vi "HatchManipulatorStateMachine.vi"(5 "Reset":bool, 6 "Place Release":bool, 7 "Floor Intake":bool, 8 "Place":bool, 9 "Slide/ No slide":bool, 10 "Feeder Station Intake":bool) -> (0 "Grip":bool, 1 "Hatch Manipulator State":T1, 2 "Extend":bool, 3 "Slide":bool)   [LabVIEW 2018]
uses:
  TypeDefs/HatchManipulatorState.ctl
  ArgosLib/Signal Processing/TypeDefs/EdgeDetector_Type.ctl
  ArgosLib/ArgosLib.lvlib
panel:
  in  "Grip Time (ms)":u32=500
  in  "Extend Time (ms)":u32=500
  in  "Slide Time (ms)":u32=500
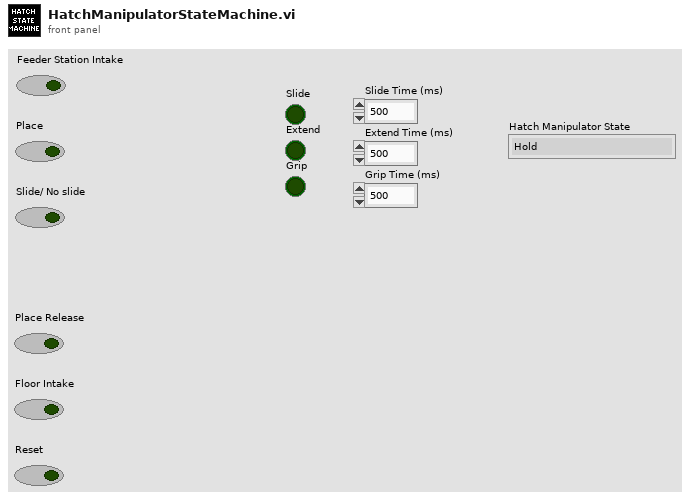
[diagram p1: front panel]
types:
  T1 = typedef "HatchManipulatorState.ctl" = enum16{"Hold", "Feeder Station Slide Out", "Feeder Station Slide Extend", "Feeder Station Slide Fully Extend", "Feeder Station Slide Grip", "Feeder Station Slide Retract", "Feeder Station Extend", "Feeder Station Fully Extended", "Feeder Station Grip", "Place Slide Out", "Place Slide Extend", "Place Slide Release", "Place Slide Retract", "Place Extend", "Place Release", "Place Retract", "Floor Intake Extend", "Floor Intake Grip"}
  T2 = typedef "ArgosLib.lvlib/EdgeDetector_Type.ctl" = enum16{"RisingEdge", "FallingEdge", "Both"}
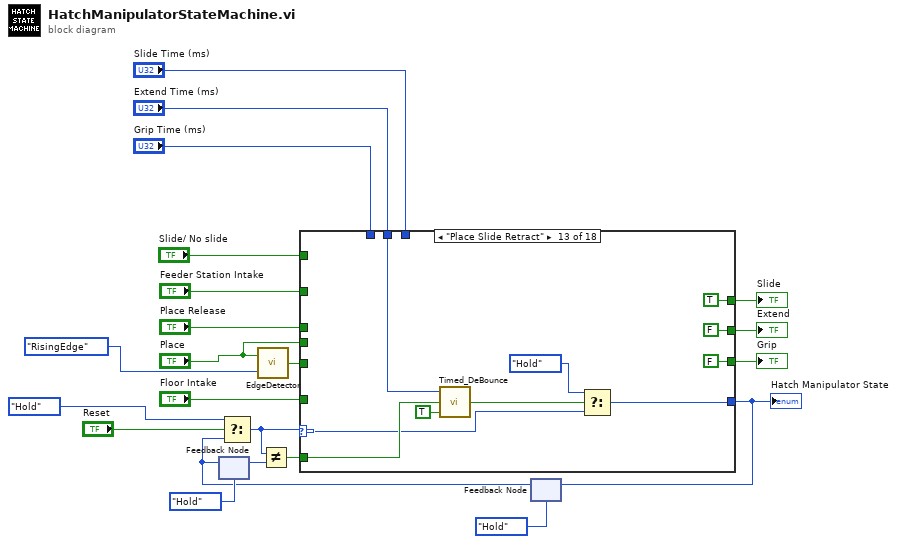
[diagram p0: block diagram]
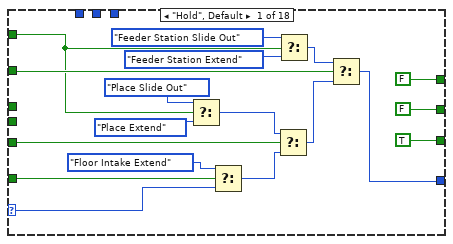
[diagram p2: hidden frame]
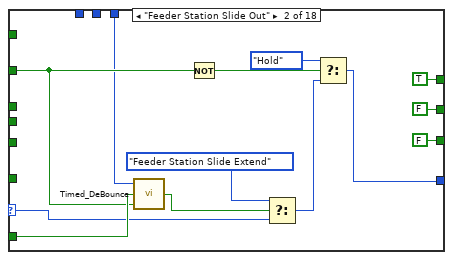
[diagram p3: hidden frame]
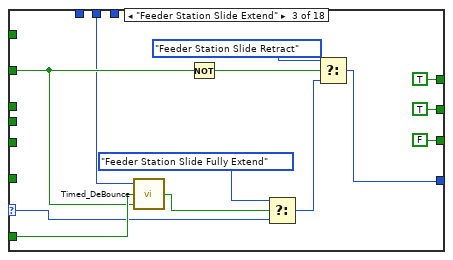
[diagram p4: hidden frame]
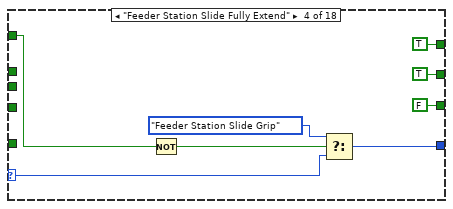
[diagram p5: hidden frame]
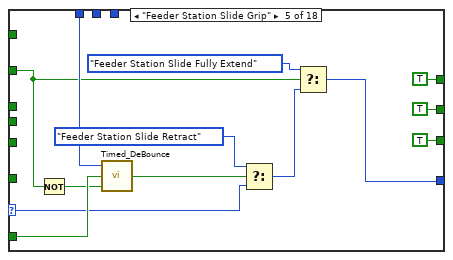
[diagram p6: hidden frame]
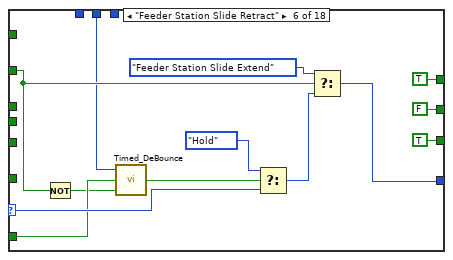
[diagram p7: hidden frame]
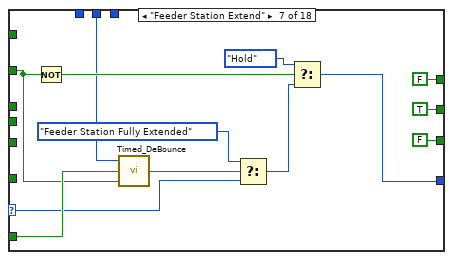
[diagram p8: hidden frame]
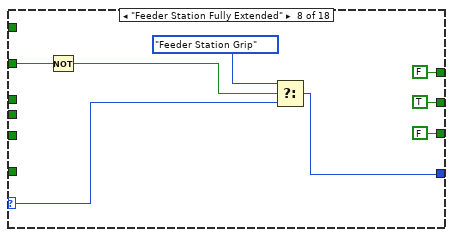
[diagram p9: hidden frame]
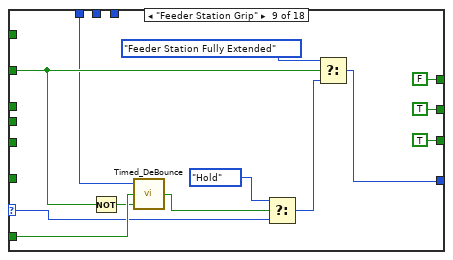
[diagram p10: hidden frame]
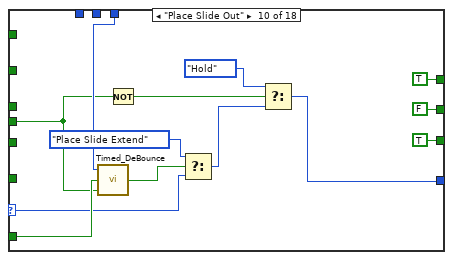
[diagram p11: hidden frame]
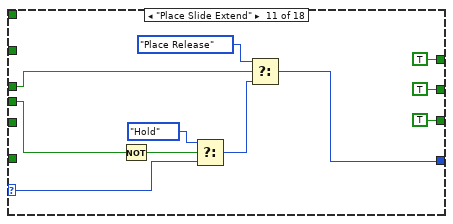
[diagram p12: hidden frame]
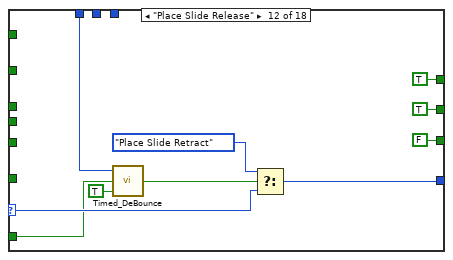
[diagram p13: hidden frame]
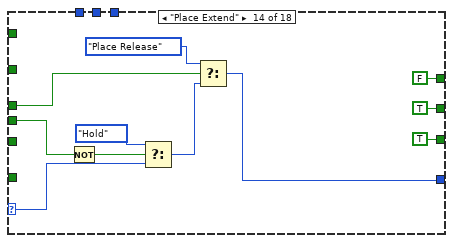
[diagram p14: hidden frame]
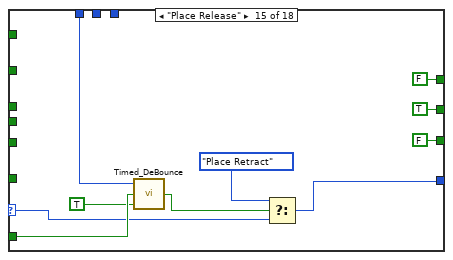
[diagram p15: hidden frame]
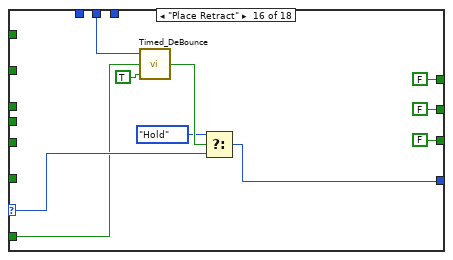
[diagram p16: hidden frame]
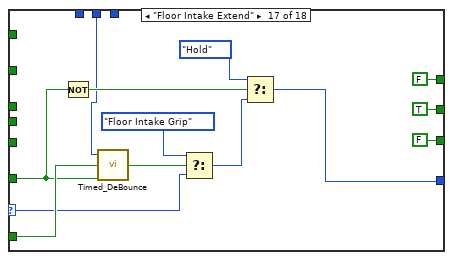
[diagram p17: hidden frame]
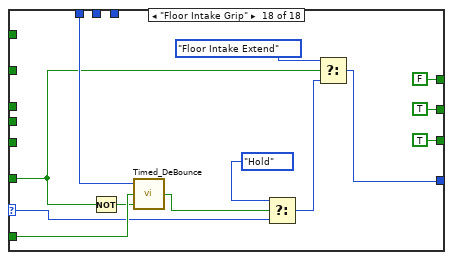
[diagram p18: hidden frame]
diagram:
  n1 = feedback #1(HatchManipulatorState."Hold" ("Hatch Manipulator State")) -> (w7:T1)
  n2 = call "EdgeDetector.vi"("DetectorType"=EdgeDetector_Type."RisingEdge", "Input"="Place") -> ("Edge"=w4:bool)
  n3 = feedback #2(HatchManipulatorState."Hold" ("Hatch Manipulator State")) -> (w8:T1)
  n4 = feedback-in #1(w8) -> ()
  n5 = Select(t=HatchManipulatorState."Hold", s="Reset", f=w8) -> (s? t:f=w9:T1)
  n6 = Not Equal?(x=w9, y=w7) -> (x != y?=w12:bool)
  n7 = case shown="\"Place Slide Retract\"" w9 {
    selector: w9 -> [w35 w46 w60 w71 w81 w93 w105 w117 w128 w141 w149 w163 w169 w186 w194 w206 w218 w230]
    tunnel: [FALSE TRUE TRUE TRUE TRUE TRUE FALSE FALSE FALSE TRUE TRUE TRUE TRUE FALSE FALSE FALSE FALSE FALSE] -> w21
    tunnel: [FALSE FALSE TRUE TRUE TRUE FALSE TRUE TRUE TRUE FALSE TRUE TRUE FALSE TRUE TRUE FALSE TRUE TRUE] -> w20
    tunnel: [TRUE FALSE FALSE FALSE TRUE TRUE FALSE FALSE TRUE TRUE TRUE FALSE FALSE TRUE FALSE FALSE FALSE TRUE] -> w19
    tunnel: "Feeder Station Intake" -> [w37 w49 w62 w69 w76 w90 w104 w118 w130 _ _ _ _ _ _ _ _ _]
    tunnel: w4 -> [w33 _ _ _ _ _ _ _ _ _ _ _ _ _ _ _ _ _]
    tunnel: "Floor Intake" -> [w36 _ _ _ _ _ _ _ _ _ _ _ _ _ _ _ w213 w223]
    tunnel: "Place Release" -> [_ _ _ _ _ _ _ _ _ _ w151 _ _ w184 _ _ _ _]
    tunnel: [w34 w42 w56 w70 w79 w89 w101 w114 w124 w139 w148 w162 w173 w180 w191 w200 w210 w226] -> w5
    tunnel: "Slide Time (ms)" -> [_ w48 _ _ _ _ _ _ _ w144 _ _ _ _ _ _ _ _]
    tunnel: "Extend Time (ms)" -> [_ _ w54 _ _ w88 w102 _ _ _ _ _ w172 _ _ w205 w211 _]
    tunnel: "Grip Time (ms)" -> [_ _ _ _ w82 _ _ _ w123 _ _ w159 _ _ w192 _ _ w225]
    tunnel: w12 -> [_ w50 w63 _ w84 w92 w106 _ w131 w143 _ w161 w171 _ w196 w204 w219 w232]
    tunnel: "Place" -> [_ _ _ _ _ _ _ _ _ w136 w150 _ _ w179 _ _ _ _]
    tunnel: "Slide/ No slide" -> [w29 _ _ _ _ _ _ _ _ _ _ _ _ _ _ _ _ _]
    frame "Hold", Default {
      n8 = Select(t=HatchManipulatorState."Place Slide Out", s=w29, f=HatchManipulatorState."Place Extend") -> (s? t:f=w26:T1)
      n9 = Select(t=HatchManipulatorState."Floor Intake Extend", s=w36, f=w35) -> (s? t:f=w31:T1)
      n10 = Select(t=w26, s=w33, f=w31) -> (s? t:f=w32:T1)
      n11 = Select(t=HatchManipulatorState."Feeder Station Slide Out", s=w29, f=HatchManipulatorState."Feeder Station Extend") -> (s? t:f=w30:T1)
      n12 = Select(t=w30, s=w37, f=w32) -> (s? t:f=w34:T1)
    }
    frame "Feeder Station Slide Out" {
      n13 = call "Timed_DeBounce.vi"("Input"=w49, "Reset"=w50, "Hold Time(ms)"=w48) -> ("Output"=w47:bool)
      n14 = Not(x=w49) -> (.not. x?=w41:bool)
      n15 = Select(t=HatchManipulatorState."Feeder Station Slide Extend", s=w47, f=w46) -> (s? t:f=w45:T1)
      n16 = Select(t=HatchManipulatorState."Hold", s=w41, f=w45) -> (s? t:f=w42:T1)
    }
    frame "Feeder Station Slide Extend" {
      n17 = call "Timed_DeBounce.vi"("Input"=w62, "Reset"=w63, "Hold Time(ms)"=w54) -> ("Output"=w61:bool)
      n18 = Not(x=w62) -> (.not. x?=w55:bool)
      n19 = Select(t=HatchManipulatorState."Feeder Station Slide Fully Extend", s=w61, f=w60) -> (s? t:f=w59:T1)
      n20 = Select(t=HatchManipulatorState."Feeder Station Slide Retract", s=w55, f=w59) -> (s? t:f=w56:T1)
    }
    frame "Feeder Station Slide Fully Extend" {
      n21 = Not(x=w69) -> (.not. x?=w67:bool)
      n22 = Select(t=HatchManipulatorState."Feeder Station Slide Grip", s=w67, f=w71) -> (s? t:f=w70:T1)
    }
    frame "Feeder Station Slide Grip" {
      n23 = Not(x=w76) -> (.not. x?=w83:bool)
      n24 = call "Timed_DeBounce.vi"("Input"=w83, "Reset"=w84, "Hold Time(ms)"=w82) -> ("Output"=w78:bool)
      n25 = Select(t=HatchManipulatorState."Feeder Station Slide Retract", s=w78, f=w81) -> (s? t:f=w80:T1)
      n26 = Select(t=HatchManipulatorState."Feeder Station Slide Fully Extend", s=w76, f=w80) -> (s? t:f=w79:T1)
    }
    frame "Feeder Station Slide Retract" {
      n27 = Not(x=w90) -> (.not. x?=w91:bool)
      n28 = call "Timed_DeBounce.vi"("Input"=w91, "Reset"=w92, "Hold Time(ms)"=w88) -> ("Output"=w96:bool)
      n29 = Select(t=HatchManipulatorState."Hold", s=w96, f=w93) -> (s? t:f=w97:T1)
      n30 = Select(t=HatchManipulatorState."Feeder Station Slide Extend", s=w90, f=w97) -> (s? t:f=w89:T1)
    }
    frame "Feeder Station Extend" {
      n31 = Not(x=w104) -> (.not. x?=w103:bool)
      n32 = call "Timed_DeBounce.vi"("Input"=w104, "Reset"=w106, "Hold Time(ms)"=w102) -> ("Output"=w109:bool)
      n33 = Select(t=HatchManipulatorState."Feeder Station Fully Extended", s=w109, f=w105) -> (s? t:f=w110:T1)
      n34 = Select(t=HatchManipulatorState."Hold", s=w103, f=w110) -> (s? t:f=w101:T1)
    }
    frame "Feeder Station Fully Extended" {
      n35 = Not(x=w118) -> (.not. x?=w115:bool)
      n36 = Select(t=HatchManipulatorState."Feeder Station Grip", s=w115, f=w117) -> (s? t:f=w114:T1)
    }
    frame "Feeder Station Grip" {
      n37 = Not(x=w130) -> (.not. x?=w122:bool)
      n38 = call "Timed_DeBounce.vi"("Input"=w122, "Reset"=w131, "Hold Time(ms)"=w123) -> ("Output"=w129:bool)
      n39 = Select(t=HatchManipulatorState."Hold", s=w129, f=w128) -> (s? t:f=w127:T1)
      n40 = Select(t=HatchManipulatorState."Feeder Station Fully Extended", s=w130, f=w127) -> (s? t:f=w124:T1)
    }
    frame "Place Slide Out" {
      n41 = call "Timed_DeBounce.vi"("Input"=w136, "Reset"=w143, "Hold Time(ms)"=w144) -> ("Output"=w142:bool)
      n42 = Not(x=w136) -> (.not. x?=w135:bool)
      n43 = Select(t=HatchManipulatorState."Place Slide Extend", s=w142, f=w141) -> (s? t:f=w140:T1)
      n44 = Select(t=HatchManipulatorState."Hold", s=w135, f=w140) -> (s? t:f=w139:T1)
    }
    frame "Place Slide Extend" {
      n45 = Not(x=w150) -> (.not. x?=w154:bool)
      n46 = Select(t=HatchManipulatorState."Hold", s=w154, f=w149) -> (s? t:f=w155:T1)
      n47 = Select(t=HatchManipulatorState."Place Release", s=w151, f=w155) -> (s? t:f=w148:T1)
    }
    frame "Place Slide Release" {
      n48 = call "Timed_DeBounce.vi"("Input"=TRUE, "Reset"=w161, "Hold Time(ms)"=w159) -> ("Output"=w165:bool)
      n49 = Select(t=HatchManipulatorState."Place Slide Retract", s=w165, f=w163) -> (s? t:f=w162:T1)
    }
    frame "Place Slide Retract" {
      n50 = call "Timed_DeBounce.vi"("Input"=TRUE, "Reset"=w171, "Hold Time(ms)"=w172) -> ("Output"=w175:bool)
      n51 = Select(t=HatchManipulatorState."Hold", s=w175, f=w169) -> (s? t:f=w173:T1)
    }
    frame "Place Extend" {
      n52 = Not(x=w179) -> (.not. x?=w181:bool)
      n53 = Select(t=HatchManipulatorState."Hold", s=w181, f=w186) -> (s? t:f=w185:T1)
      n54 = Select(t=HatchManipulatorState."Place Release", s=w184, f=w185) -> (s? t:f=w180:T1)
    }
    frame "Place Release" {
      n55 = call "Timed_DeBounce.vi"("Input"=TRUE, "Reset"=w196, "Hold Time(ms)"=w192) -> ("Output"=w195:bool)
      n56 = Select(t=HatchManipulatorState."Place Retract", s=w195, f=w194) -> (s? t:f=w191:T1)
    }
    frame "Place Retract" {
      n57 = call "Timed_DeBounce.vi"("Input"=TRUE, "Reset"=w204, "Hold Time(ms)"=w205) -> ("Output"=w202:bool)
      n58 = Select(t=HatchManipulatorState."Hold", s=w202, f=w206) -> (s? t:f=w200:T1)
    }
    frame "Floor Intake Extend" {
      n59 = Not(x=w213) -> (.not. x?=w212:bool)
      n60 = call "Timed_DeBounce.vi"("Input"=w213, "Reset"=w219, "Hold Time(ms)"=w211) -> ("Output"=w214:bool)
      n61 = Select(t=HatchManipulatorState."Floor Intake Grip", s=w214, f=w218) -> (s? t:f=w217:T1)
      n62 = Select(t=HatchManipulatorState."Hold", s=w212, f=w217) -> (s? t:f=w210:T1)
    }
    frame "Floor Intake Grip" {
      n63 = Not(x=w223) -> (.not. x?=w224:bool)
      n64 = call "Timed_DeBounce.vi"("Input"=w224, "Reset"=w232, "Hold Time(ms)"=w225) -> ("Output"=w231:bool)
      n65 = Select(t=HatchManipulatorState."Hold", s=w231, f=w230) -> (s? t:f=w229:T1)
      n66 = Select(t=HatchManipulatorState."Floor Intake Extend", s=w223, f=w229) -> (s? t:f=w226:T1)
    }
  }
  "Slide" <- w21
  "Extend" <- w20
  "Grip" <- w19
  "Hatch Manipulator State" <- w5
  n67 = feedback-in #2(w5) -> ()
